vi "Different Signs.vi"(8 "error in (no error)":errorcluster, 10 "High Res Arithmetic In 2":refnum<class "Rational Number.lvclass">, 11 "High Res Arithmetic In":refnum<class "Rational Number.lvclass">) -> (0 "error out":errorcluster, 2 "Different signs?":bool)   [LabVIEW 2021, in "Rational Number.lvclass"]
uses:
  High Res Arithmetic/Rational Number.lvclass
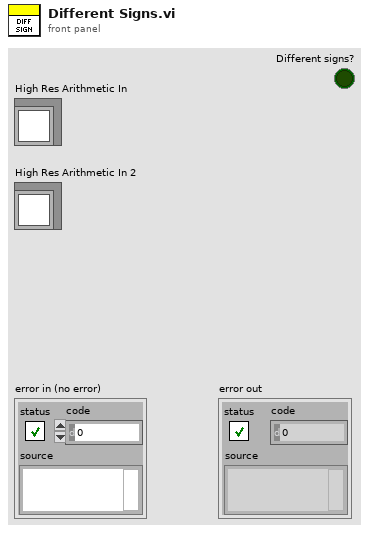
[diagram p1: front panel]
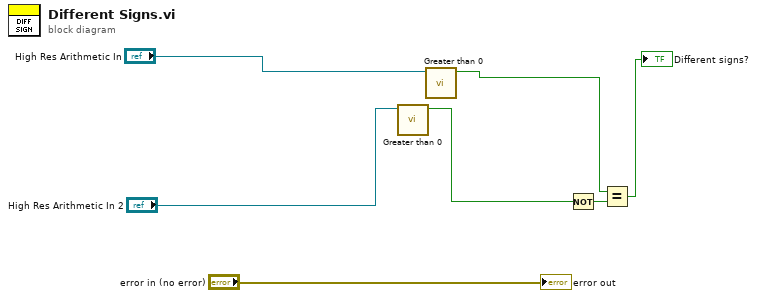
[diagram p0: block diagram]
diagram:
  n1 = call "Greater than 0.vi"("Rational Number in"="High Res Arithmetic In 2") -> ("Greater than 0?"=w4:bool)  [unwired: 10 in]
  n2 = call "Greater than 0.vi"("Rational Number in"="High Res Arithmetic In") -> ("Greater than 0?"=w1:bool)  [unwired: 10 in]
  n3 = Not(x=w4) -> (.not. x?=w3:bool)
  n4 = Equal?(x=w1, y=w3) -> (x = y?=→"Different signs?":bool)
  "error out" <- "error in (no error)"
